vi "IT6322_Measure.vi"(7 "等待时间(毫秒)":u32=100, 8 "error in":errorcluster caption="错误输入（无错误）", 9 "CH":enum16{"CH1", "CH2", "CH3"}(ring), 10 "Measure":T1(ring), 11 "MyIndex":u8) -> (0 "error out":errorcluster, 2 "数值":dbl, 3 "状态":bool)   [LabVIEW 2015, in "IT6322.lvlib"]
uses:
  IT6322.lvlib
  <vilib>/Instr/_visa.llb/VISA Configure Serial Port (Instr).vi
panel:
  out "返回值":string
  out "VISA":refnum<visa-resource-name>
  out "数组":dbl[](array[numeric])
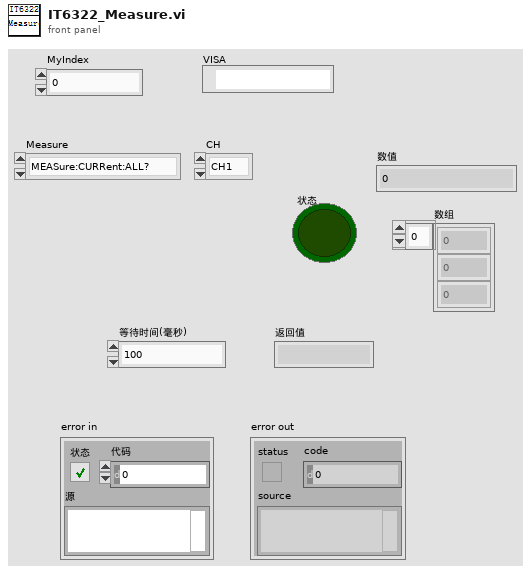
[diagram p1: front panel]
types:
  T1 = enum16{"MEASure:CURRent:ALL?", "MEASure:VOLTage:ALL?"}
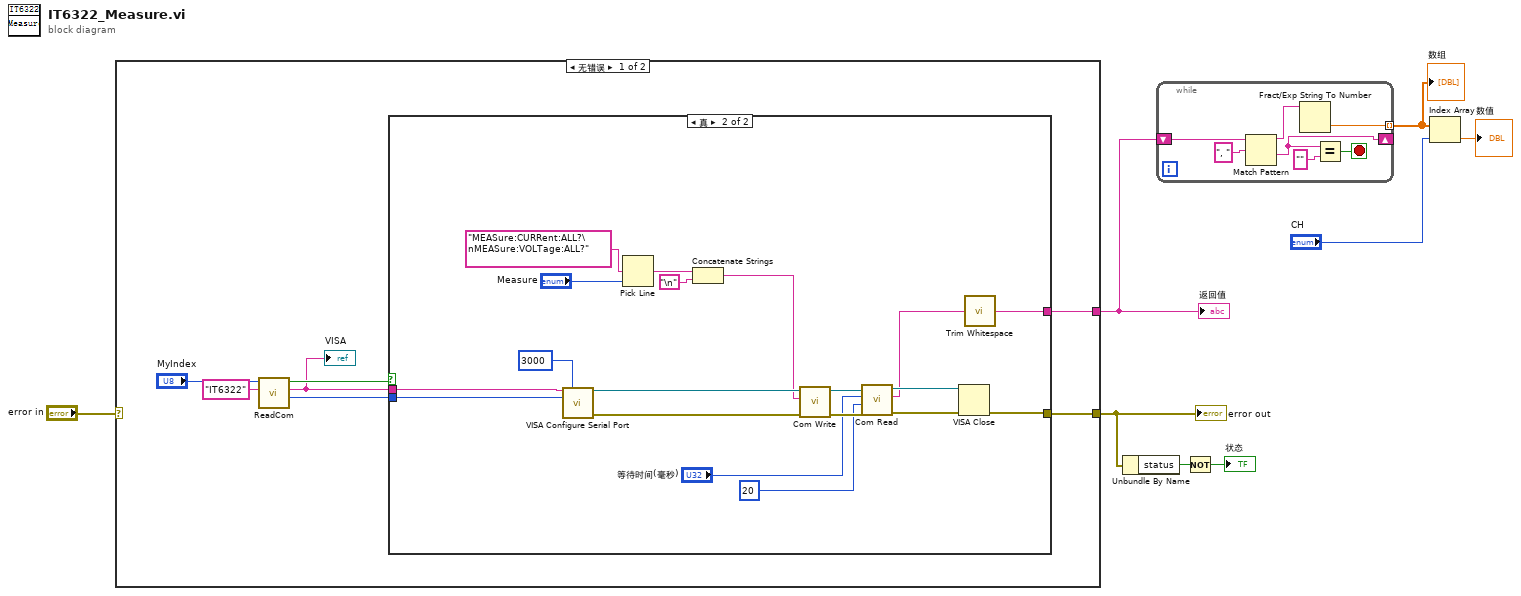
[diagram p0: block diagram]
diagram:
  n1 = case shown="无错误" "error in" {
    selector: "error in" -> [_ w35]
    tunnel: [w15 w35] -> w3
    tunnel: [w9 _] -> w1
    frame No Error {
      n2 = call "ReadCom.vi"("仪器名称"="IT6322", "MyIndex"="MyIndex") -> ("Baudrate"=w10:i32, "COM"=w11:string, "OK?"=w12:bool)  [unwired: 7 in]
      "VISA" <- w11
      n3 = case shown="真" w12 {
        tunnel: [_ w34] -> w15
        tunnel: w11 -> [_ w33]
        tunnel: w10 -> [_ w32]
        tunnel: [_ w16] -> w9
        frame False {
        }
        frame True {
          n4 = call-poly "VISA Configure Serial Port"("VISA resource name"=w33, "timeout (10sec)"=u32 3000, "baud rate (9600)"=w32) -> ("VISA resource name out"=w30:refnum<visa-resource-name>, "error out"=w29:errorcluster)  [unwired: 11 in]
          n5 = Pick Line(multi-line string="MEASure:CURRent:ALL?\nMEASure:VOLTage:ALL?", line index="Measure") -> (output string=w21:string)  [unwired: 1 in]
          n6 = Concatenate Strings(w21, "\n") -> (w17:string)
          n7 = call "Com Write.vi"("错误输入（无错误）"=w29, "Wbuff"=w17, "VISA In"=w30) -> ("错误输出"=w27:errorcluster, "VISA Out"=w28:refnum<visa-resource-name>)  [unwired: 7 in]
          n8 = call "Com Read.vi"("错误输入（无错误）"=w27, "num"=u32 20, "超时"="等待时间(毫秒)", "VISA In"=w28) -> ("错误输出"=w26:errorcluster, "buff"=w24:string, "VISA Out"=w25:refnum<visa-resource-name>)  [unwired: 5 in]
          n9 = VISA Close(VISA resource name=w25, error in (no error)=w26) -> (error out=w34:errorcluster)
          n10 = call <vilib>:"Trim Whitespace.vi"("string"=w24) -> ("trimmed string"=w16:string)  [unwired: 1 in]
        }
      }
    }
    frame Error {
    }
  }
  "error out" <- w3
  "返回值" <- w1
  n11 = Unbundle By Name(w3) -> ("status"=w2:bool)
  n12 = while {
    shift-right: [w39] -> _
    shift-left: w1 -> [w38]
    tunnel: [w36] -> w8 mode=indexing
    stop <- w40 stop-if-true
    n13 = Match Pattern(string=w38, regular expression=", " ("正则表达式")) -> (before substring=w37:string, after substring=w39:string)  [unwired: 1 in, 2 out]
    n14 = Fract/Exp String To Number(string=w37) -> (number=w36:dbl)  [unwired: 3 in, 1 out]
    n15 = Equal?(x=w39, y="") -> (x = y?=w40:bool)
  }
  "数组" <- w8
  n16 = Not(x=w2) -> (.not. x?=→"状态":bool)
  n17 = Index Array(array=w8, index="CH") -> (element=→"数值":dbl)
